vi "Write Get Connection List Msg.vi"(10 "Connection Handler.lvlib:Get Connection List Msg.lvclass":refnum<class "Get Connection List Msg.lvclass">=refnum, 11 "Connection Handler in":refnum<class "Connection Handler.lvclass">) -> (3 "Connection Handler out":refnum<class "Connection Handler.lvclass">)   [LabVIEW 2017]
uses:
  Connection Handler.lvclass
  Volumes/Data/Users/benji667/Git/BuildFarm/WebSocket Server/Actors/Actor wHelper/Actor wHelper/Actor wHelper.lvclass
  Volumes/Data/Users/benji667/Git/BuildFarm/WebSocket Server/Actors/Actor wHelper/Actor wLauncher/Actor wLauncher.lvclass
  Volumes/Data/Users/benji667/Git/BuildFarm/WebSocket Server/Actors/Actor wHelper/Actor wUI/Actor wUI.lvclass
  Applications/National Instruments/LabVIEW 2017 64-bit/vi.lib/ActorFramework/Actor/Actor.lvclass
  Connection Handler Messages/Get Connection List Msg/Get Connection List Msg.lvclass
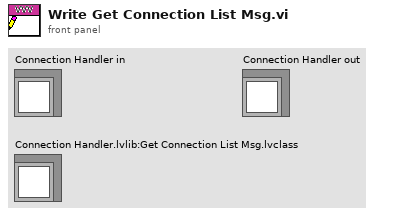
[diagram p1: front panel]
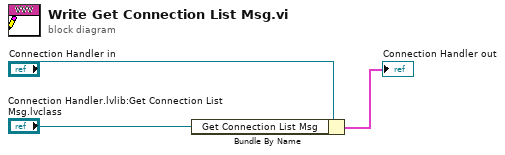
[diagram p0: block diagram]
diagram:
  n1 = Bundle By Name(cluster="Connection Handler in", "Get Connection List Msg"="Connection Handler.lvlib:Get Connection List Msg.lvclass") -> (→"Connection Handler out":cluster{})
